vi "ConvertProjectConditionalDeactivationValuesKeys.vi"(8 "Fehler (Eingang, kein Fehler)":errorcluster, 10 "CondDeact":cluster{"Keys":string[], "Values":string[]}) -> (0 "Fehler (Ausgang)":errorcluster, 2 "Tabellen-String":string)   [LabVIEW 2020, in "ConditionalDeactivation.lvlib"]
uses:
  ConditionalDeactivation.lvlib
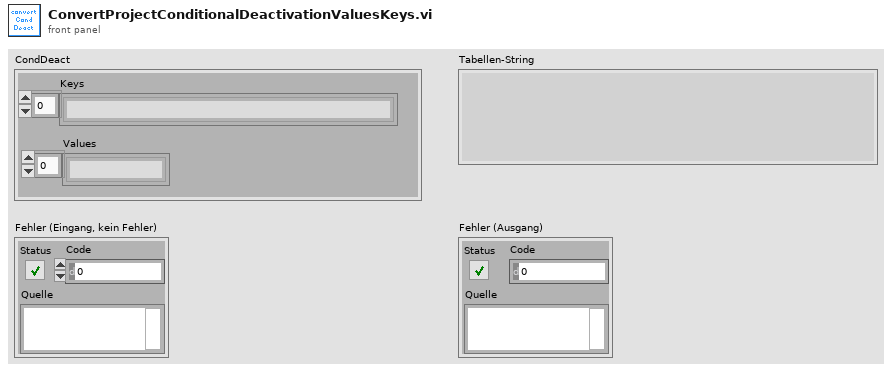
[diagram p1: front panel]
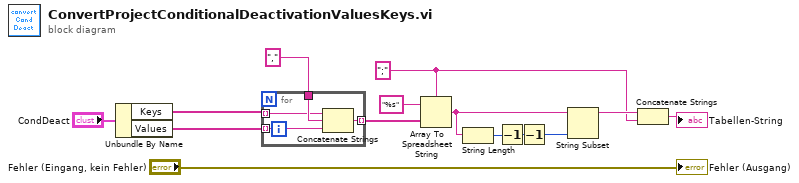
[diagram p0: block diagram]
diagram:
  w1 = ";" ("Trennzeichen (Tabulator)")
  n1 = Unbundle By Name("CondDeact") -> ("Keys"=w13:string[], "Values"=w12:string[])
  n2 = for {
    tunnel: w13 -> [w17] mode=indexing
    tunnel: w12 -> [w15] mode=indexing
    tunnel: "," ("String") -> [w18]
    tunnel: [w16] -> w11 mode=indexing
    n3 = Concatenate Strings(w17, w18, w15) -> (w16:string)
  }
  n4 = Array To Spreadsheet String(delimiter (Tab)=w1, array=w11, 3:"%s" ("Format-String")) -> (spreadsheet string=w5:string)
  n5 = String Length(string=w5) -> (length=w6:i32)
  n6 = Decrement(x=w6) -> (x-1=w4:i32)
  n7 = Decrement(x=w4) -> (x-1=w3:i32)
  n8 = String Subset(string=w5, length (rest)=w3) -> (substring=w7:string)  [unwired: 1 in]
  n9 = Concatenate Strings(w7, w1) -> (→"Tabellen-String":string)
  "Fehler (Ausgang)" <- "Fehler (Eingang, kein Fehler)"
